vi "VI Analyzer Project Provider User Guide.vi"   [LabVIEW 2015]
uses:
  <vilib>/Platform/browser.llb/Open URL in Default Browser (path).vi
panel:
  # "Opening User Guide...."
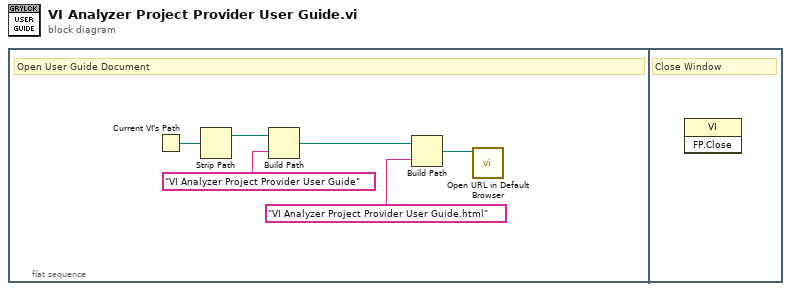
[diagram p0: block diagram]
diagram:
  n1 = flat-sequence {
    frame #0 {
      # "Open User Guide Document"
      n2 = Current VI's Path() -> (path=w6:path)
      n3 = Strip Path(path=w6) -> (stripped path=w5:path)  [unwired: 1 out]
      n4 = Build Path(base path=w5, name or relative path="VI Analyzer Project Provider User Guide") -> (appended path=w4:path)
      n5 = Build Path(base path=w4, name or relative path="VI Analyzer Project Provider User Guide.html") -> (appended path=w3:path)
      n6 = call-poly <vilib>:"Open URL in Default Browser.vi"("path"=w3) -> ()  [unwired: 5 in, 2 out]
    }
    frame #1 {
      # "Close Window"
      n7 = invoke class="VI" method="FP.Close"() -> ()  [unwired: 3 in, 3 out]
    }
  }
